vi "Runtime Test.vi"() -> ()   [LabVIEW 2014, in "UI Reference tests.lvlib"]
doc: "This VI shows an example for how to test the Runtime functionality of the module. This will need to be modified according to module functionality."
uses:
  UI Reference tests.lvlib
  module/execution/UI Reference runtime.lvclass
  <vilib>/NI/Tag Bus/dictionary/data dictionary.lvclass/data dictionary.ctl
  <vilib>/NI/Tag Bus/dictionary/lookup polymorphs/locate double.vi
  <vilib>/NI/Tag Bus/table/data polymorphs/read one/read Double.vi
  <vilib>/NI/Tag Bus/table/data polymorphs/write one/write Double.vi
  <vilib>/NI/Tag Bus/dictionary/search/find data index.vi
  <vilib>/NI/Tag Bus/dictionary/search/search string list.vi
  <vilib>/NI/Tag Bus/dictionary/tag not found.vi
  module/configuration/UI Reference configuration.lvclass
  <vilib>/NI/Tag Bus/dictionary/data dictionary.lvclass
  <vilib>/NI/Tag Bus/table/data table.lvlib
panel:
  out "Names":string[](array[string])
  out "Input":dbl
  in  "output value":dbl=42.0 format="%#_13g"
  out "error":errorcluster
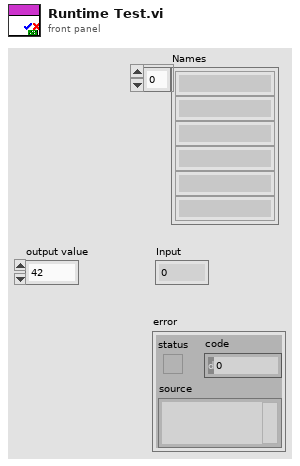
[diagram p1: front panel]
types:
  T1 = typedef "TBM channel.lvclass/data tables.ctl" = cluster{"input data":T2, "processing parameter":T2, "processing result":T2, "output data":T2}
  T2 = typedef "tag bus.lvlib/dictionary table pair.ctl" = cluster{"data dictionary":refnum<class "data dictionary.lvclass">, "data table":T3}
  T3 = typedef "tag bus.lvlib/data table.lvlib/data table.ctl" = cluster{"Double":dbl[], "Single":sgl[], "I64":i64[], "I32":i32[], "I16":i16[], "I8":i8[], "U64":u64[], "U32":u32[], "U16":u16[], "U8":u8[], "Boolean":bool[], "String":string[], "Array of Double":cluster{"DBL Array":dbl[]}[], "Array of Single":cluster{"SGL Array":sgl[]}[], "Array of I64":cluster{"I64 Array":i64[]}[], "Array of I32":cluster{"I32 Array":i32[]}[], "Array of I16":cluster{"I16 Array":i16[]}[], "Array of I8":cluster{"I8 Array":i8[]}[], "Array of U64":cluster{"U64 Array":u64[]}[], "Array of U32":cluster{"U32 Array":u32[]}[], "Array of U16":cluster{"U16 Array":u16[]}[], "Array of U8":cluster{"U8 Array":u8[]}[], "Array of Boolean":cluster{"Boolean Array":bool[]}[], "Array of String":cluster{"String Array":string[]}[]}
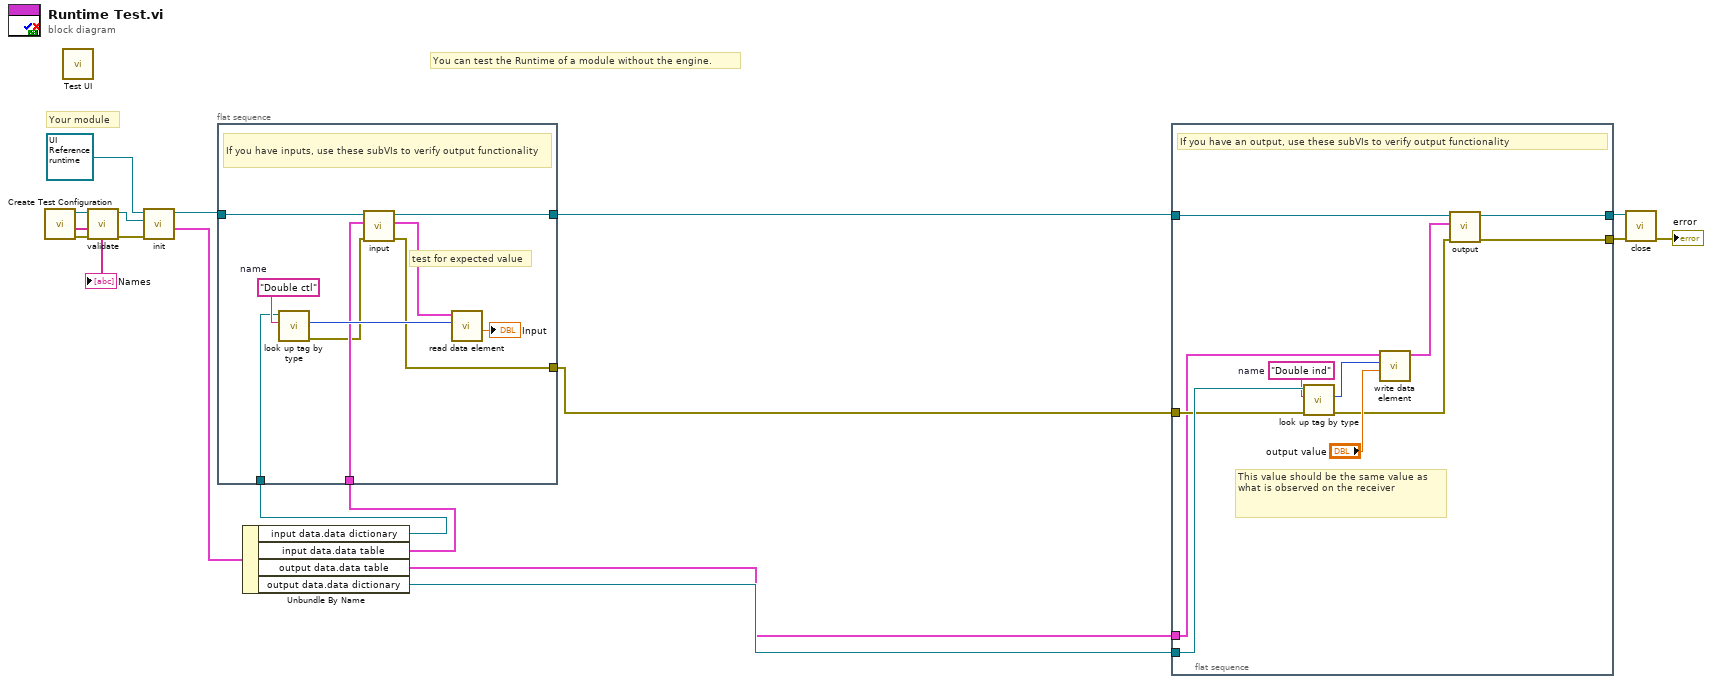
[diagram p0: block diagram]
diagram:
  # "You can test the Runtime of a module without the engine."
  # "Your module"
  n1 = call "Create Test Configuration.vi"() -> ("error out"=w13:errorcluster, "Names"=→"Names":string[], "Module Configuration"=w14:refnum<class "UI Reference configuration.lvclass">)  [unwired: 6 in, 3 out]
  n2 = call "Test UI.vi"() -> ()  [unwired: 12 in]
  n3 = call-dynamic "validate.vi"("error in"=w13, "UI Reference configuration in"=w14) -> ("error out"=w16:errorcluster, "UI Reference configuration out"=w15:refnum<class "UI Reference configuration.lvclass">)  [unwired: 8 in]
  n4 = call-dynamic "init.vi"("error in"=w16, "TBM module configuration in"=w15, "UI Reference runtime in"=refnum<class "UI Reference runtime.lvclass"> refnum ("tag bus configurable plugin module")) -> ("data allocations"=w4:T1, "UI Reference runtime out"=w5:refnum<class "UI Reference runtime.lvclass">)  [unwired: 5 in, 2 out]
  n5 = flat-sequence {
    tunnel: [w20] -> w2
    tunnel: w5 -> [w27]
    tunnel: [w26] -> w3
    tunnel: w7 -> [w24]
    tunnel: w6 -> [w21]
    frame #0 {
      w25 = "Double ctl"  # name
      # "test for expected value"
      # "If you have inputs, use these subVIs to verify output functionality"
      n6 = call-poly <vilib>:"look up tag by type.vi"("name"=w25, "data dictionary in"=w24) -> ("error out"=w19:errorcluster, "index"=w22:i32)  [unwired: 7 in, 1 out]
      n7 = call-dynamic "input.vi"("error in"=w19, "data table in"=w21, "UI Reference runtime in"=w27) -> ("error out"=w20:errorcluster, "data table out"=w23:T3, "UI Reference runtime out"=w26:refnum<class "UI Reference runtime.lvclass">)  [unwired: 6 in]
      n8 = call-poly <vilib>:"read data element.vi"("index"=w22, "data table in"=w23) -> ("value"=→"Input":dbl)  [unwired: 8 in, 1 out]
    }
  }
  n9 = Unbundle By Name(w4) -> ("input data.data dictionary"=w7:refnum<class "data dictionary.lvclass">, "input data.data table"=w6:T3, "output data.data table"=w8:T3, "output data.data dictionary"=w12:refnum<class "data dictionary.lvclass">)
  n10 = flat-sequence {
    tunnel: w12 -> [w38]
    tunnel: [w34] -> w11
    tunnel: [w33] -> w10
    tunnel: w3 -> [w32]
    tunnel: w2 -> [w31]
    tunnel: w8 -> [w30]
    frame #0 {
      w28 = "Double ind"  # name
      # "This value should be the same value as what is observed on the receiver"
      # "If you have an output, use these subVIs to verify output functionality"
      n11 = call-poly <vilib>:"look up tag by type.vi"("error in"=w31, "name"=w28, "data dictionary in"=w38) -> ("error out"=w29:errorcluster, "index"=w37:i32)  [unwired: 6 in, 1 out]
      n12 = call-poly <vilib>:"write data element.vi"("value"="output value", "index"=w37, "data table in"=w30) -> ("data table out"=w35:T3)  [unwired: 8 in]
      n13 = call-dynamic "output.vi"("error in"=w29, "data table in"=w35, "UI Reference runtime in"=w32) -> ("error out"=w33:errorcluster, "UI Reference runtime out"=w34:refnum<class "UI Reference runtime.lvclass">)  [unwired: 6 in, 1 out]
    }
  }
  n14 = call-dynamic "close.vi"("error in"=w10, "UI Reference runtime in"=w11) -> ("error out"=→"error":errorcluster)  [unwired: 9 in]
